vi "is_initialized.vi"(8 "error in (no error)":errorcluster, 11 "FPGAWrapperMH120124RAPS_PXI7813R in":refnum<class "FPGAWrapperMH120124RAPS_PXI7813R.lvclass">) -> (0 "error out":errorcluster, 2 "is initialized?":bool, 3 "FPGAWrapperMH120124RAPS_PXI7813R out":refnum<class "FPGAWrapperMH120124RAPS_PXI7813R.lvclass">)   [LabVIEW 2010, in "FPGAWrapperMH120124RAPS_PXI7813R.lvclass"]
uses:
  FPGAWrapperMH120124RAPS_PXI7813R.lvclass
  class_data.vi
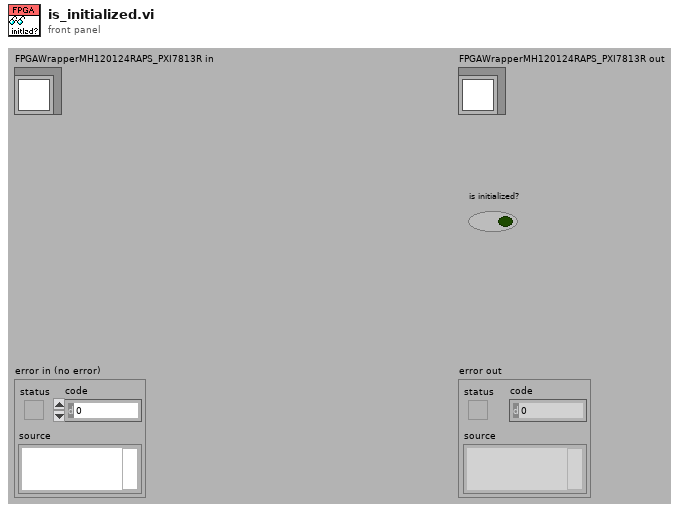
[diagram p1: front panel]
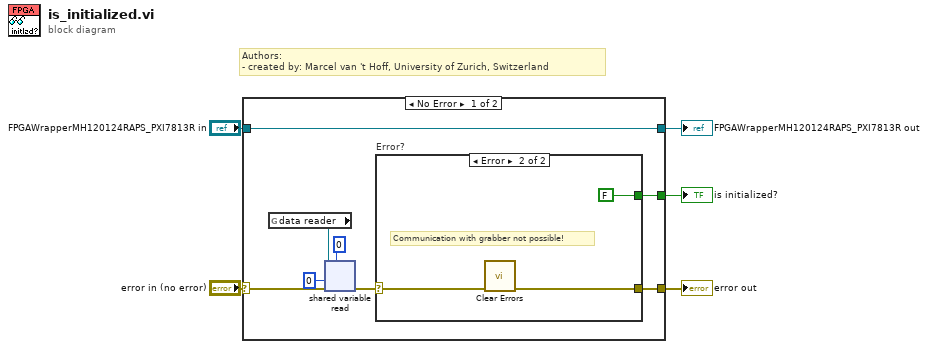
[diagram p0: block diagram]
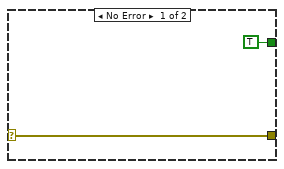
[diagram p2: hidden frame]
diagram:
  # "Authors: \n- created by: Marcel van 't Hoff, University of Zurich, Switzerland"
  n1 = case shown="No Error" "error in (no error)" {
    selector: "error in (no error)" -> [w9 w20]
    tunnel: [w8 w20] -> w4
    tunnel: [w13 w19] -> w2
    tunnel: "FPGAWrapperMH120124RAPS_PXI7813R in" -> [w13 w19]
    tunnel: [w7 _] -> w1
    frame No Error {
      n2 = global read "class_data.vi" "data reader"() -> (w6:refnum<k21>)
      n3 = shared-variable-read(w6, w9, 0 ("timeout in ms (-1)"), 0 ("# elements (-1)")) -> (w12:errorcluster)  [unwired: 3 out]
      n4 = case "Error?" shown="Error" w12 {
        selector: w12 -> [w15 w17]
        tunnel: [TRUE FALSE] -> w7
        tunnel: [w15 w16] -> w8
        frame No Error {
        }
        frame Error {
          # "Communication with grabber not possible!"
          n5 = call <vilib>:"Clear Errors.vi"("error in (no error)"=w17) -> ("error out"=w16:errorcluster)  [unwired: 6 in]
        }
      }
    }
    frame Error {
    }
  }
  "error out" <- w4
  "FPGAWrapperMH120124RAPS_PXI7813R out" <- w2
  "is initialized?" <- w1
